vi "Test App Removed Process Lifecycle Not Managed by App.vi"(8 "error in (no error)":errorcluster, 11 "Rig Test in":refnum<class "Application Test.lvclass">) -> (0 "error out":errorcluster, 3 "Rig Test out":refnum<class "Application Test.lvclass">)   [LabVIEW 2020, in "Application Test.lvclass"]
uses:
  Application Test.lvclass
  C:/Program Files (x86)/National Instruments/LabVIEW 2020/vi.lib/Asteme/LUnit/Test Case.lvclass
  Framework/Process/Process.lvclass
  Framework/Process/Public/Lifecycle/Lifecycle State.ctl
  Framework/Process/Process.lvclass/Process.ctl
  Framework/Application/Application.lvclass/Application.ctl
  <vilib>/Asteme/LUnit/Test Case.lvclass/Test Case.ctl
  <vilib>/Asteme/LUnit/LUnit Assertion Result.lvclass/LUnit Assertion Result.ctl
  Framework/Application/Private/Add Process to Map.vi
  Framework/Application/Private/Start Idle Processes if Running.vi
  Framework/Process/Protected/Messaging/Enqueue Message.vi
  Framework/Process/Protected/SubVIs/Set Context.vi
  Framework/Process/Private/SubVIs/Wait for finish.vi
  Framework/Process/Private/SubVIs/Set Lifecycle State.vi
  <vilib>/Utility/error.llb/Clear Errors.vi
  <vilib>/Asteme/LUnit/Palette/Fail.vi
  <vilib>/Asteme/LUnit/Palette/Pass.vi
  <vilib>/Asteme/LUnit/Set Assertion Type.vi
  Framework/Process/Public/Lifecycle/Leave Process Loop.vi
  <vilib>/Asteme/LUnit/Add test result.vi
  <vilib>/Asteme/LUnit/LUnit Write Passed.vi
  <vilib>/Asteme/LUnit/LUnit Get Test Case.vi
  <vilib>/Asteme/LUnit/Assertion Result/LUnit Get Test Name.vi
  <vilib>/Asteme/LUnit/LUnit Write Message.vi
  <vilib>/Asteme/LUnit/LUnit Write Description.vi
  <vilib>/Asteme/LUnit/LUnit Write Assertion Type.vi
  <vilib>/Asteme/LUnit/Read Test Case Name.vi
  Framework/Application/Application.lvclass
  C:/Users/anton/Documents/GitHub/Triarc-Framework/source/Framework/Process/Process.lvclass
  <vilib>/Utility/error.llb/Error Cluster From Error Code.vi
  Framework/Application/Private/Throw Error If Process Already in App.vi
  Framework/Process/Public/Read Name.vi
  Framework/Application/Private/Update Context for Owned Processes.vi
  <vilib>/Asteme/LUnit/LUnit Assertion Result.lvclass
  <vilib>/Asteme/LUnit/Test Case.lvclass
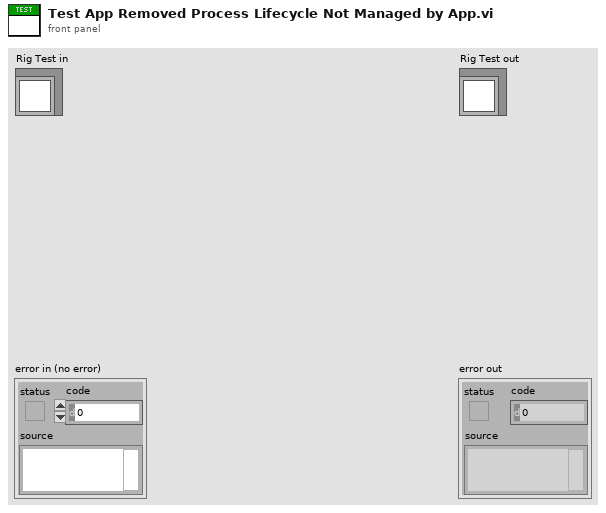
[diagram p1: front panel]
types:
  T1 = typedef "Process.lvclass/Lifecycle State.ctl" = enum16{"Uninitialized", "Initialized", "Started", "Running", "Stopped", "Finished"}
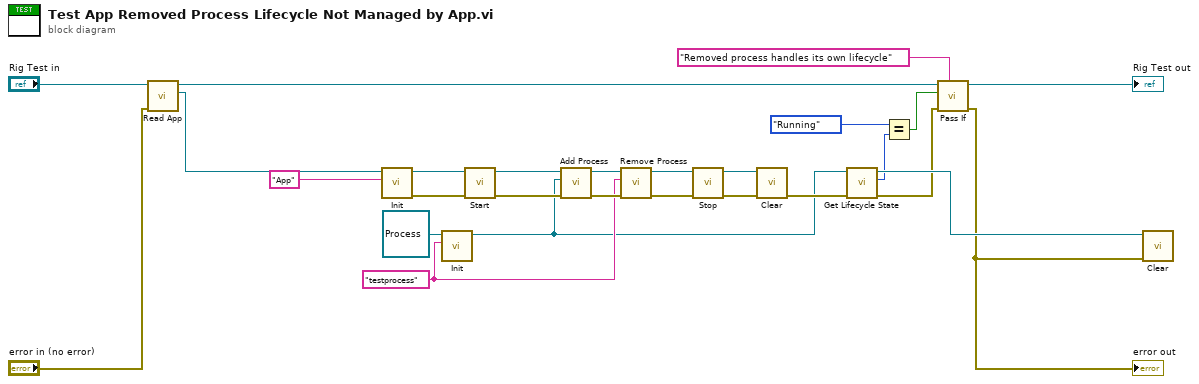
[diagram p0: block diagram]
diagram:
  w8 = "testprocess" ("Name")
  n1 = call "Read App.vi"("error in (no error)"="error in (no error)", "Application Test In"="Rig Test in") -> ("App out"=w26:refnum<class "Application.lvclass">, "Application Test Out"=w17:refnum<class "Application Test.lvclass">)  [unwired: 7 in, 1 out]
  n2 = call-dynamic "Init.vi"("Name"="App", "Process In"=w26) -> ("error out"=w18:errorcluster, "Process Out"=w19:refnum<class "Application.lvclass">)  [unwired: 8 in]
  n3 = call-dynamic "Init.vi"("Name"=w8, "Process In"=refnum<class "Process.lvclass"> refnum ("Process.lvclass")) -> ("Process Out"=w1:refnum<class "Process.lvclass">)  [unwired: 8 in, 1 out]
  n4 = call "Start.vi"("error in (no error)"=w18, "Process In"=w19) -> ("error out"=w20:errorcluster, "Process Out"=w10:refnum<class "Application.lvclass">)  [unwired: 7 in, 1 out]
  n5 = call "Add Process.vi"("error in (no error)"=w20, "Process"=w1, "Rig In"=w10) -> ("error out"=w23:errorcluster, "Rig Out"=w12:refnum<class "Application.lvclass">)  [unwired: 7 in]
  n6 = call "Remove Process.vi"("error in (no error)"=w23, "Process Name"=w8, "Rig In"=w12) -> ("error out"=w13:errorcluster, "Rig Out"=w11:refnum<class "Application.lvclass">)  [unwired: 6 in, 1 out]
  n7 = call "Stop.vi"("error in (no error)"=w13, "Process In"=w11) -> ("error out"=w15:errorcluster, "Process Out"=w14:refnum<class "Application.lvclass">)  [unwired: 7 in, 1 out]
  n8 = call-dynamic "Clear.vi"("error in (no error)"=w15, "Application In"=w14) -> ("error out"=w9:errorcluster)  [unwired: 9 in]
  n9 = call "Get Lifecycle State.vi"("error in (no error)"=w9, "Process In"=w1) -> ("error out"=w6:errorcluster, "Lifecycle State"=w4:T1, "Process Out"=w7:refnum<class "Process.lvclass">)  [unwired: 6 in, 1 out]
  n10 = Equal?(x=Lifecycle_State."Running" ("Lifecycle State"), y=w4) -> (x = y?=w2:bool)
  n11 = call <vilib>:"Pass If.vi"("Description"="Removed process handles its own lifecycle", "error in (no error)"=w6, "Pass?"=w2, "Test Case In"=w17) -> ("error out"=w5:errorcluster, "Test Case Out"=→"Rig Test out":refnum<class "Application Test.lvclass">)  [unwired: 6 in]
  "error out" <- w5
  n12 = call-dynamic "Clear.vi"("error in (no error)"=w5, "Process In"=w7) -> ()  [unwired: 9 in, 1 out]
